vi "UPS Variable.vi"() -> ()   [LabVIEW 2010]
panel:
  out "UPS Array":dbl[](array[numeric])
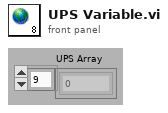
[diagram p1: front panel]
diagram:
